vi "parseTimestamp.vi"(8 "error in (no error)":errorcluster, 11 "FrameParser in":refnum<class "DynamicFrameParser.lvclass">) -> (0 "error out":errorcluster, 2 "Timestamp":dbl, 3 "FrameParser out":refnum<class "DynamicFrameParser.lvclass">)   [LabVIEW 2016, in "DynamicFrameParser.lvclass"]
uses:
  DynamicFrameParser.lvclass
  DynamicFrameParser.lvclass/DynamicFrameParser.ctl
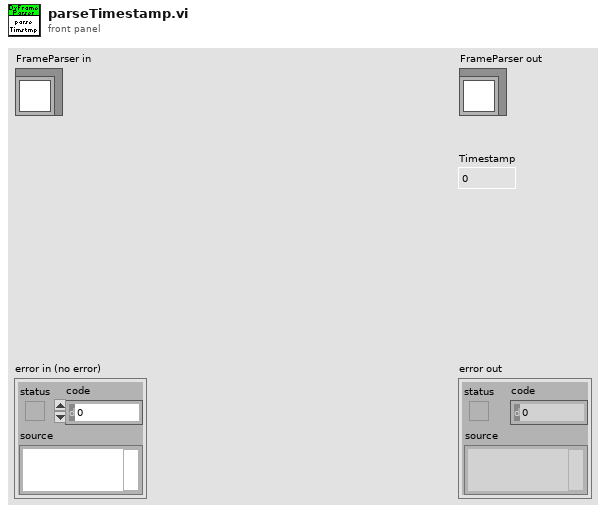
[diagram p1: front panel]
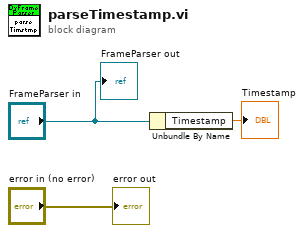
[diagram p0: block diagram]
diagram:
  n1 = Unbundle By Name("FrameParser in") -> ("Timestamp"=→"Timestamp":dbl)
  "error out" <- "error in (no error)"
  "FrameParser out" <- "FrameParser in"
